vi "XY sorter (SubVI).vi"(10 "I (A)":dbl[](array[numeric]), 11 "V (Volt)":dbl[](array[numeric])) -> (1 "sorted I (A)":dbl[](array[numeric]), 2 "sorted V (Volt)":dbl[](array[numeric]))   [LabVIEW 2014]
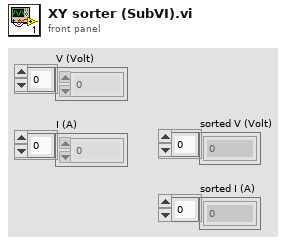
[diagram p1: front panel]
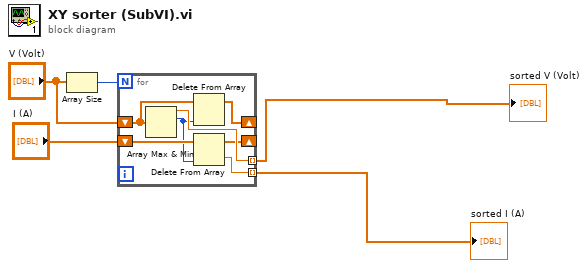
[diagram p0: block diagram]
diagram:
  n1 = Array Size(array="V (Volt)") -> (size(s)=w5:i32)
  n2 = for {
    N: w5 -> [_]
    shift-right: [w11] -> _
    shift-left: "V (Volt)" -> [w12]
    shift-right: [w7] -> _
    shift-left: "I (A)" -> [w9]
    tunnel: [w10] -> w2 mode=indexing
    tunnel: [w6] -> w1 mode=indexing
    n3 = Array Max & Min(array=w12) -> (max value=w10:dbl, max index (indices)=w8:i32)  [unwired: 2 out]
    n4 = Delete From Array(array=w12, index=w8) -> (array with subset deleted=w11:dbl[])  [unwired: 1 in, 1 out]
    n5 = Delete From Array(array=w9, index=w8) -> (deleted portion=w6:dbl, array with subset deleted=w7:dbl[])  [unwired: 1 in]
  }
  "sorted I (A)" <- w1
  "sorted V (Volt)" <- w2
